vi "selectData.vi"(8 "error in (no error)":errorcluster, 10 "SQL query":string, 11 "sqlerver in":refnum<class "sqlerver.lvclass">) -> (0 "error out":errorcluster, 1 "data":string[][](array[string]), 3 "sqlerver out":refnum<class "sqlerver.lvclass">)   [LabVIEW 2016, in "sqlerver.lvclass"]
uses:
  sqlerver.lvclass
  sqlerver.lvclass/sqlerver.ctl
  <vilib>/addons/database/Connection.llb/Conn Execute.vi
  <vilib>/addons/database/Recordset.llb/Rec Fetch Recordset Data (R).vi
  <vilib>/addons/database/Recordset.llb/Rec Destroy - Connection.vi
  <vilib>/addons/database/_DB Variant To Data/Database Variant To Data.xnode
  <vilib>/addons/database/NI_Database_API.lvlib
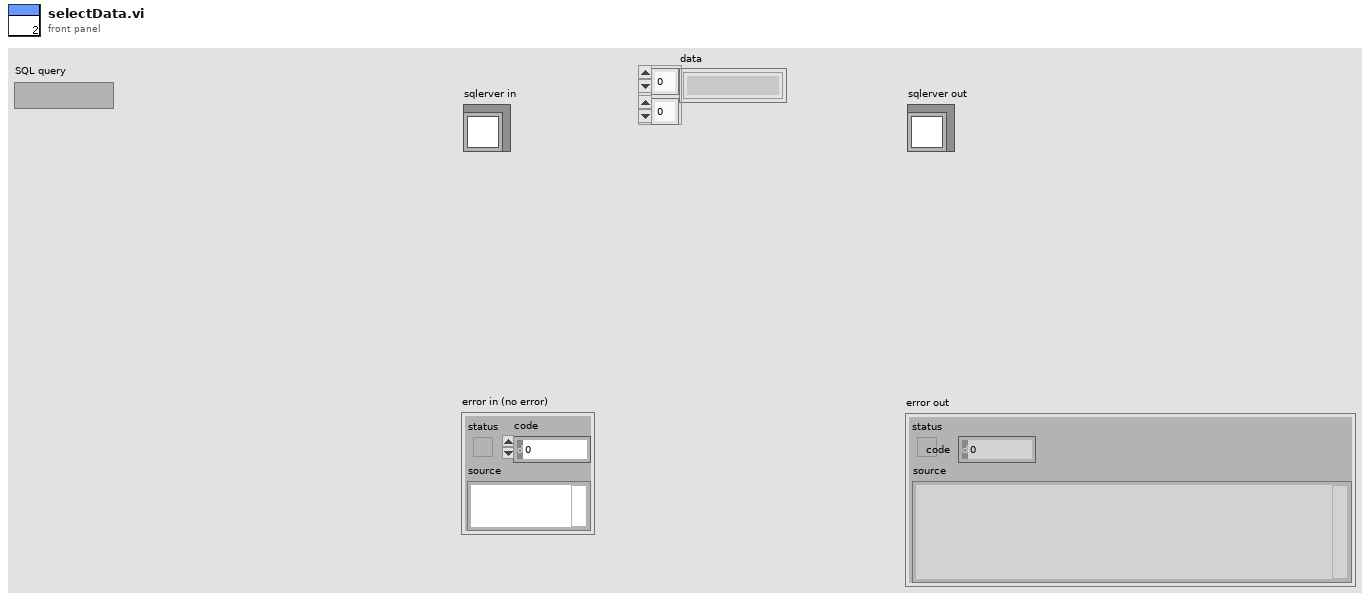
[diagram p1: front panel]
types:
  T1 = typedef "NI_Database_API.lvlib/Conn ObjectReference.ctl" = refnum<k1>
  T2 = typedef "NI_Database_API.lvlib/Rec ObjectReference.ctl" = refnum<k1>
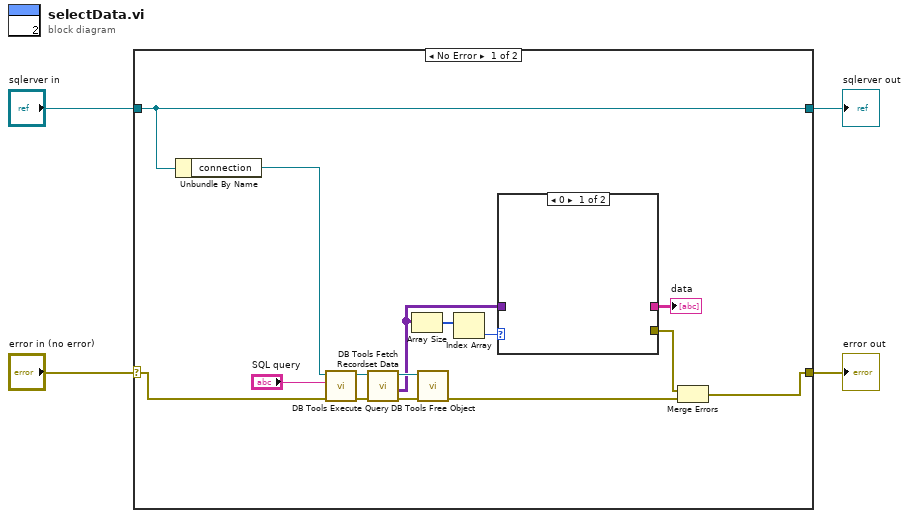
[diagram p0: block diagram]
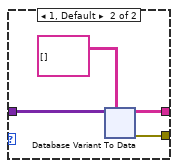
[diagram p2: hidden frame]
diagram:
  n1 = case shown="No Error" "error in (no error)" {
    selector: "error in (no error)" -> [w7 w69]
    tunnel: [w6 w69] -> w3
    tunnel: [w19 w68] -> w1
    tunnel: "sqlerver in" -> [w19 w68]
    frame No Error {
      n2 = Unbundle By Name(w19) -> ("connection"=w5:T1)
      n3 = call-poly <vilib>:"DB Tools Execute Query.vi"("error in (no error)"=w7, "SQL query"="SQL query", "connection reference"=w5) -> ("error out"=w18:errorcluster, "recordset reference"=w17:T2)  [unwired: 5 in]
      n4 = call-poly <vilib>:"DB Tools Fetch Recordset Data.vi"("error in (no error)"=w18, "recordset reference"=w17) -> ("error out"=w15:errorcluster, "recordset data"=w11:variant[][], "recordset reference out"=w16:T2)  [unwired: 3 in]
      n5 = Array Size(array=w11) -> (size(s)=w10:i32[])
      n6 = call-poly <vilib>:"DB Tools Free Object.vi"("error in (no error)"=w15, "recordset reference"=w16) -> ("error out"=w14:errorcluster)  [unwired: 8 in, 1 out]
      n7 = Index Array(array=w10) -> (element=w9:i32)  [unwired: 1 in]
      n8 = case shown="0" w9 {
        tunnel: [_ w23] -> w13
        tunnel: w11 -> [_ w22]
        tunnel: [_ w20] -> w8
        frame 0 {
        }
        frame 1, Default {
          n9 = xnode "Database Variant To Data"("database variant"=w22, "type"=string[][] []) -> ("data"=w20:string[][], "error out"=w23:errorcluster)  [unwired: 1 in]
        }
      }
      "data" <- w8
      n10 = Merge Errors(w13, w14) -> (w6:errorcluster)
    }
    frame Error {
    }
  }
  "error out" <- w3
  "sqlerver out" <- w1
